vi "centered_gaussian_3(SubVI).vi"(6 "time":dbl, 7 "Frequency(MHz)":dbl, 8 "Pulse Lenth (us)":dbl format="%#_13g", 9 "Pulse Center":dbl=5.0 format="%#_13g", 10 "Envelope DecayTime(micro s)":dbl, 11 "Amplitude":dbl) -> (3 "output":dbl)   [LabVIEW 2016]
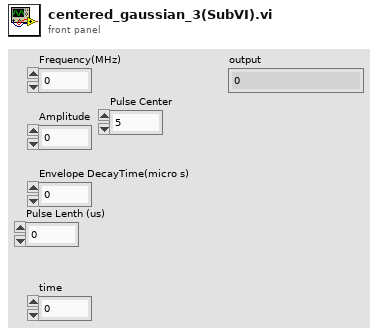
[diagram p1: front panel]
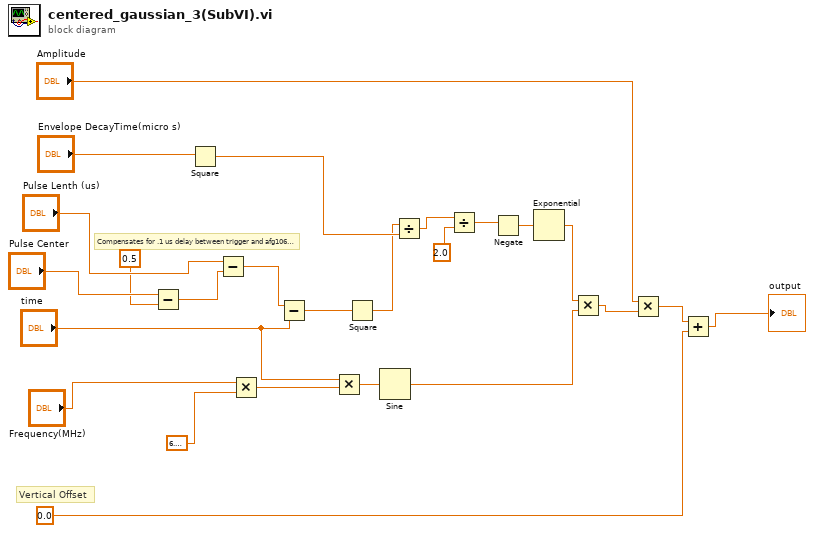
[diagram p0: block diagram]
diagram:
  # "Vertical Offset"
  # "Compensates for .1 us delay between trigger and afg1062 responding"
  n1 = Subtract(x="Pulse Center", y=0.5) -> (x-y=w7:dbl)
  n2 = Square(x="Envelope DecayTime(micro s)") -> (x^2=w15:dbl)
  n3 = Subtract(x="Pulse Lenth (us)", y=w7) -> (x-y=w6:dbl)
  n4 = Multiply(x="Frequency(MHz)", y=6.283185307179586) -> (x*y=w13:dbl)
  n5 = Subtract(x=w6, y="time") -> (x-y=w12:dbl)
  n6 = Multiply(x="time", y=w13) -> (x*y=w20:dbl)
  n7 = Square(x=w12) -> (x^2=w14:dbl)
  n8 = Sine(x=w20) -> (sin(x)=w18:dbl)
  n9 = Divide(x=w14, y=w15) -> (x/y=w22:dbl)
  n10 = Divide(x=w22, y=2.0) -> (x/y=w21:dbl)
  n11 = Negate(x=w21) -> (-x=w16:dbl)
  n12 = Exponential(1:w16) -> (0:w17:dbl)
  n13 = Multiply(x=w17, y=w18) -> (x*y=w25:dbl)
  n14 = Multiply(x="Amplitude", y=w25) -> (x*y=w3:dbl)
  n15 = Add(x=w3, y=0.0) -> (x+y=→"output":dbl)
